vi "Remote_call_prep.vi"(3 "Vi Name in":string, 4 "Job Directory In":path, 5 "VI Directory":path) -> (0 "Vi Name out":string, 1 "Job Directory out":path, 2 "cancelled":bool)   [LabVIEW 2010]
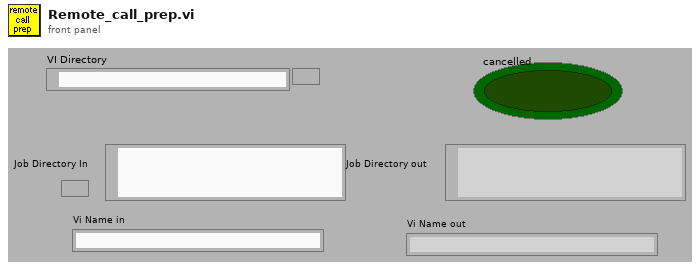
[diagram p1: front panel]
types:
  T1 = enum16{"Zero or one", "One", "Zero or more", "One or more"}
  T2 = enum32{"existing file", "new file", "new or existing file", "existing dir", "new dir", "new or existing dir", "existing file (use LLBs)", "new file (use LLBs)", "new or existing file (use LLBs)", "new or existing file or directory (use LLBs)"}
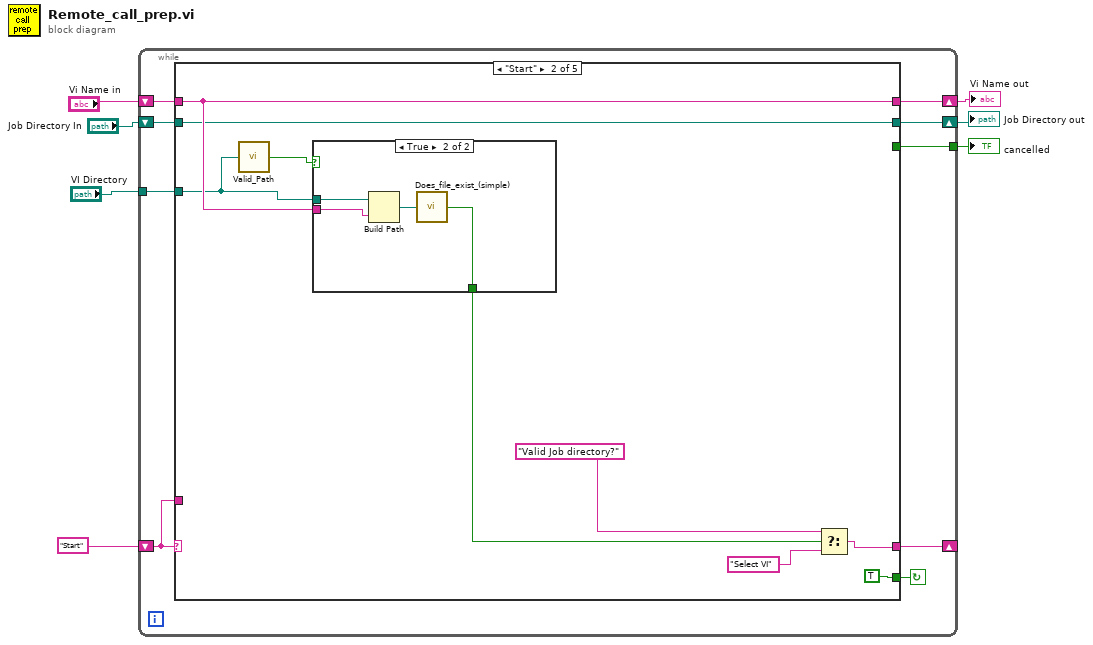
[diagram p0: block diagram]
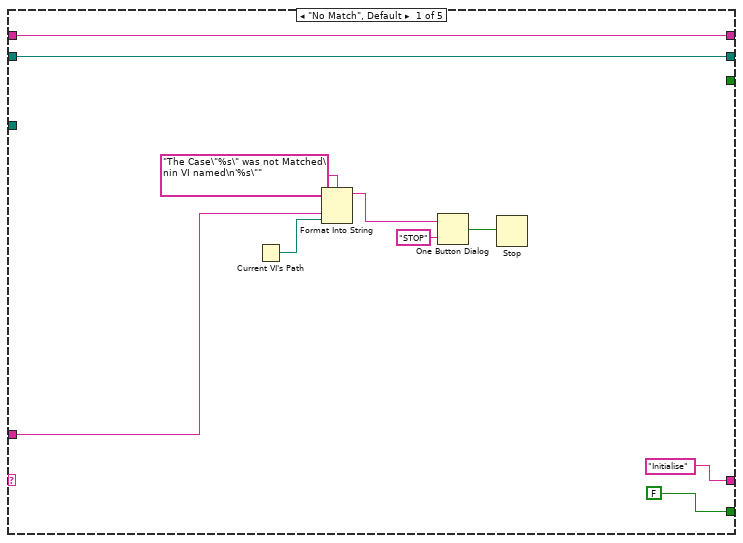
[diagram p2: hidden frame]
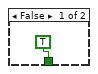
[diagram p3: hidden frame]
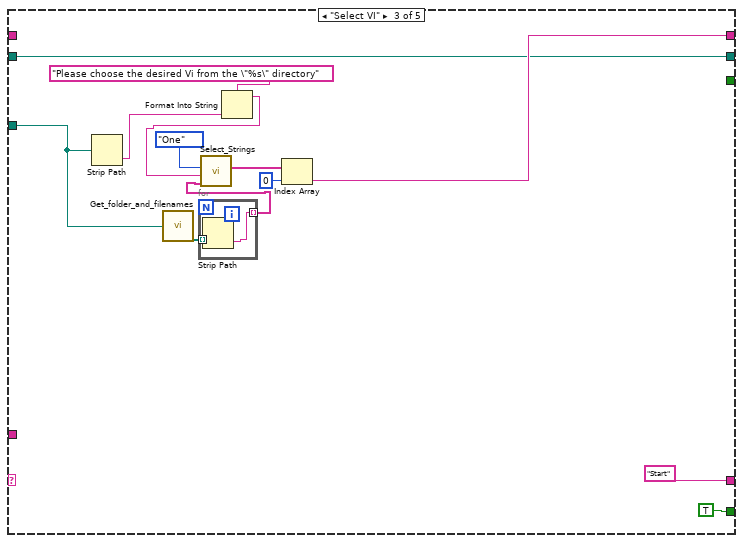
[diagram p4: hidden frame]
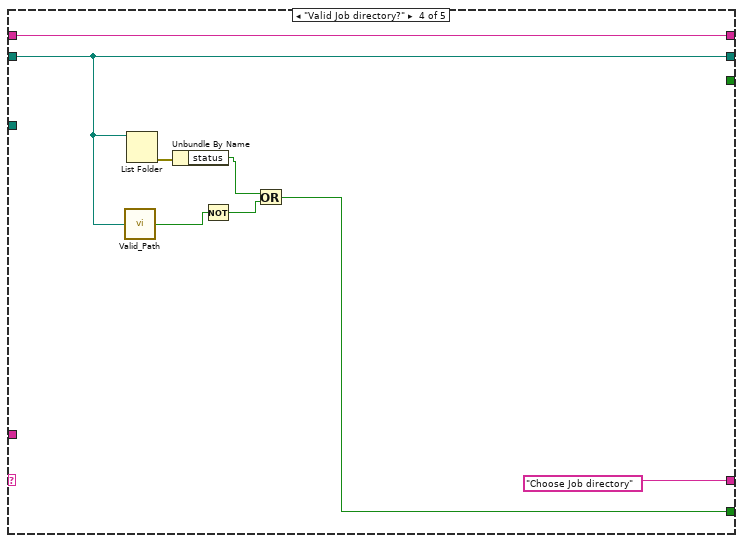
[diagram p5: hidden frame]
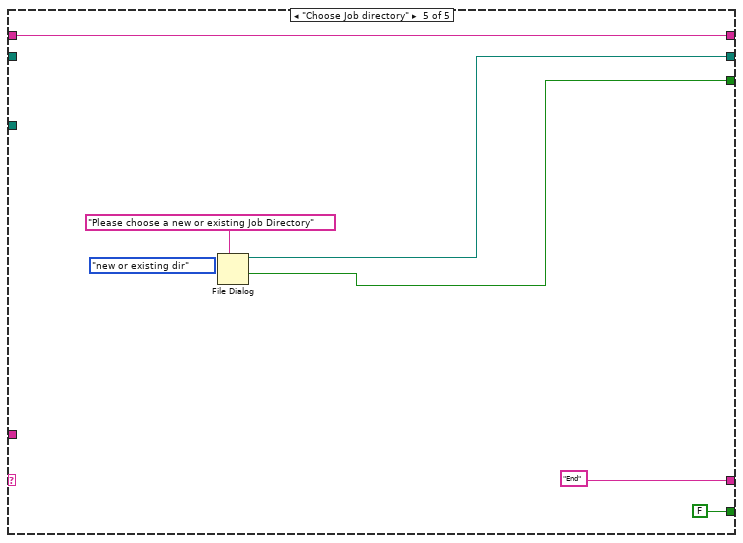
[diagram p6: hidden frame]
diagram:
  n1 = while {
    shift-left: "Start" -> [w14]
    shift-right: [w15] -> _
    tunnel: "VI Directory" -> [w13]
    shift-right: [w11] -> w4
    shift-left: "Vi Name in" -> [w12]
    shift-right: [w9] -> w1
    shift-left: "Job Directory In" -> [w10]
    tunnel: [w8] -> w2
    stop <- w16 continue-if-true
    n2 = case shown="\"Start\"" w14 {
      tunnel: [FALSE TRUE TRUE w60 FALSE] -> w16
      tunnel: ["Initialise" w31 "Start" "Choose Job directory" "End"] -> w15
      tunnel: w14 -> [w21 _ _ _ _]
      tunnel: w13 -> [_ w28 w44 _ _]
      tunnel: w12 -> [w18 w30 _ w61 w69]
      tunnel: [w18 w30 w46 w61 w69] -> w11
      tunnel: w10 -> [w17 w29 w45 w58 _]
      tunnel: [w17 w29 w45 w58 w67] -> w9
      tunnel: [_ _ _ _ w66] -> w8
      frame "No Match", Default {
        n3 = Current VI's Path() -> (path=w20:path)
        n4 = Format Into String(format string="The Case\"%s\" was not Matched\nin VI named\n'%s\"" ("Format String"), w21, w20) -> (resulting string=w24:string)  [unwired: 2 in, 1 out]
        n5 = One Button Dialog(message=w24, button name ("OK")="STOP") -> (true=w22:bool)
        n6 = Stop(stop? (T)=w22) -> ()
      }
      frame "Start" {
        n7 = call "Valid_Path.vi"("Filename"=w28) -> ("Valid Path?"=w27:bool)
        n8 = case shown="True" w27 {
          tunnel: [TRUE ("exists?") w39] -> w34
          tunnel: w30 -> [_ w38]
          tunnel: w28 -> [_ w37]
          frame False {
          }
          frame True {
            n9 = Build Path(base path=w37, name or relative path=w38) -> (appended path=w40:path)
            n10 = call "Does_file_exist_(simple).vi"("Pathname"=w40) -> ("exists?"=w39:bool)
          }
        }
        n11 = Select(t="Valid Job directory?", s=w34, f="Select VI") -> (s? t:f=w31:string)
      }
      frame "Select VI" {
        n12 = Strip Path(path=w44) -> (name=w43:string)  [unwired: 1 out]
        n13 = call "Get_folder_and_filenames.vi"("file path (dialog if empty)"=w44) -> ("Files"=w50:path[])  [unwired: 1 out]
        n14 = for {
          tunnel: w50 -> [w55] mode=indexing
          tunnel: [w54] -> w51 mode=indexing
          n15 = Strip Path(path=w55) -> (name=w54:string)  [unwired: 1 out]
        }
        n16 = Format Into String(format string="Please choose the desired Vi from the \"%s\" directory" ("Message"), w43) -> (resulting string=w41:string)  [unwired: 2 in, 1 out]
        n17 = call "Select_Strings.vi"("Available Ch names"=w51, "Message"=w41, "Selector mode"=T1."One") -> ("Selected Channel Names"=w48:string[])  [unwired: 1 in, 4 out]
        n18 = Index Array(array=w48, index=0) -> (element=w46:string)
      }
      frame "Valid Job directory?" {
        n19 = call "Valid_Path.vi"("Filename"=w58) -> ("Valid Path?"=w57:bool)
        n20 = List Folder(path=w58) -> (error out=w63:errorcluster)  [unwired: 1 in, 5 out]
        n21 = Unbundle By Name(w63) -> ("status"=w62:bool)
        n22 = Not(x=w57) -> (.not. x?=w56:bool)
        n23 = Or(x=w62, y=w56) -> (x .or. y?=w60:bool)
      }
      frame "Choose Job directory" {
        (unwired) T2."new or existing dir" ("select mode (2)")
        n24 = File Dialog(7:"Please choose a new or existing Job Directory" ("prompt")) -> (1:w66:bool, 3:w67:path)  [unwired: 1 in, 7 out]
      }
    }
  }
  "Vi Name out" <- w4
  "cancelled" <- w2
  "Job Directory out" <- w1
